vi "Create.vi"(8 "error in (no error)":errorcluster, 9 "offset":i32, 10 "Input":string) -> (0 "error out":errorcluster, 3 "Proto":refnum<class "Proto.lvclass">)   [LabVIEW 2021, in "Proto.lvclass"]
uses:
  Proto.lvclass
  Proto.lvclass/Proto.ctl
  Helpers/Helpers.lvlib
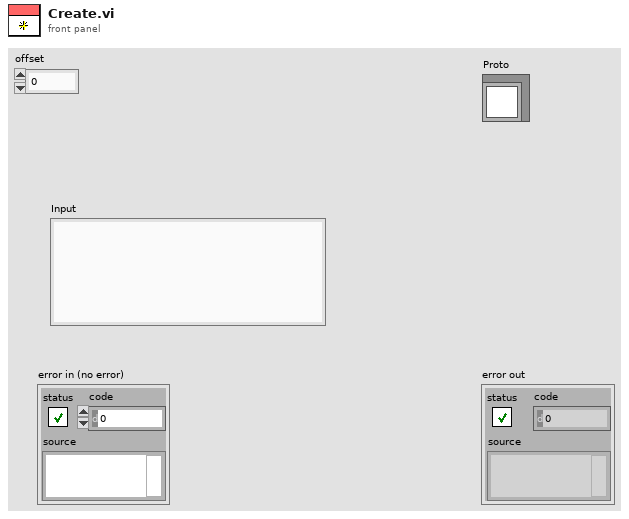
[diagram p1: front panel]
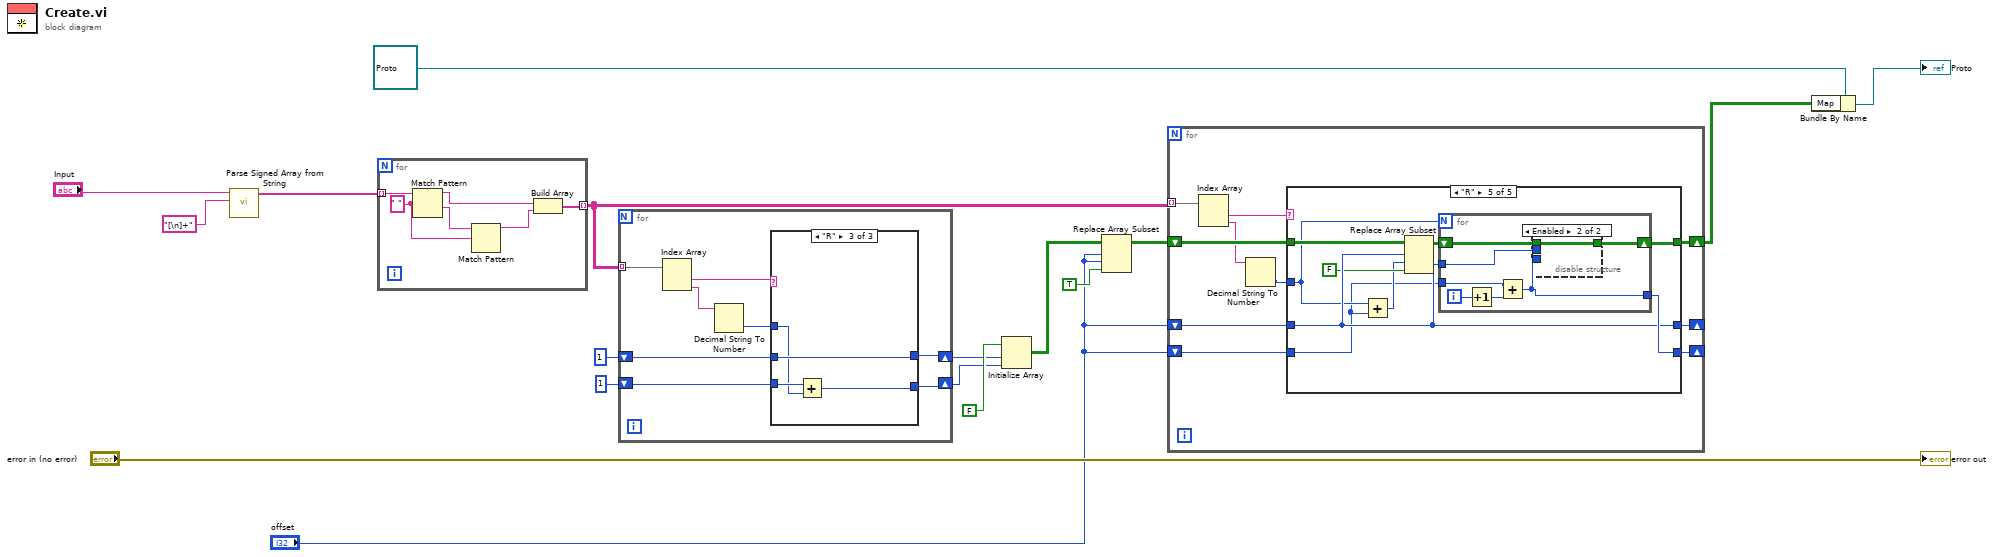
[diagram p0: block diagram]
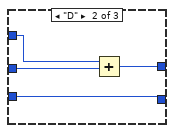
[diagram p3: hidden frame]
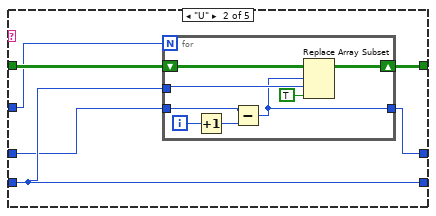
[diagram p5: hidden frame]
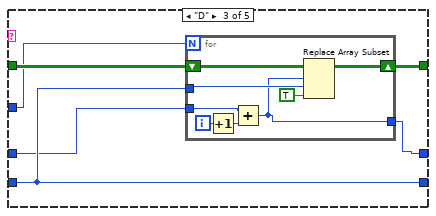
[diagram p6: hidden frame]
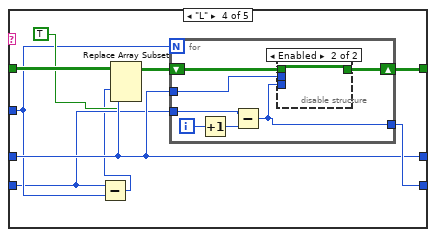
[diagram p7: hidden frame]
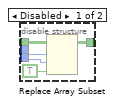
[diagram p8: hidden frame]
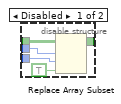
[diagram p9: hidden frame]
diagram:
  n1 = call "Parse Signed Array from String.vi"("Delimiter regex"="[\n]+", "Input"="Input") -> ("Parsed Array"=w13:string[])  [unwired: 8 in, 1 out]
  n2 = for {
    tunnel: w13 -> [w23] mode=indexing
    tunnel: [w18] -> w3 mode=indexing
    w22 = " " ("regular expression")
    n3 = Match Pattern(string=w23, regular expression=w22) -> (before substring=w19:string, after substring=w21:string)  [unwired: 1 in, 2 out]
    n4 = Match Pattern(string=w21, regular expression=w22) -> (before substring=w20:string)  [unwired: 1 in, 3 out]
    n5 = Build Array(w19, w20) -> (w18:string[])
  }
  n6 = for {
    tunnel: w3 -> [w31] mode=indexing
    shift-right: [w24] -> w8
    shift-left: 1 -> [w25]
    shift-right: [w26] -> w9
    shift-left: 1 -> [w27]
    n7 = Index Array(array=w31) -> (element #1=w30:string, element #2=w29:string)  [unwired: 2 in]
    n8 = Decimal String To Number(string=w29) -> (number=w28:i32)  [unwired: 2 in, 1 out]
    n9 = case shown="\"R\"" w30 {
      tunnel: w28 -> [_ w37 w38]
      tunnel: w27 -> [w33 w36 w41]
      tunnel: [w33 w35 w41] -> w26
      tunnel: w25 -> [w32 w34 w40]
      tunnel: [w32 w34 w39] -> w24
      frame Default {
      }
      frame "D" {
        n10 = Add(x=w37, y=w36) -> (x+y=w35:i32)
      }
      frame "R" {
        n11 = Add(x=w40, y=w38) -> (x+y=w39:i32)
      }
    }
  }
  n12 = Initialize Array(FALSE, w9, w8) -> (w6:bool[][])
  n13 = Replace Array Subset(array=w6, new element=TRUE ("new element/subarray"), index (row)="offset", index (col)="offset") -> (w5:bool[][])
  n14 = for {
    tunnel: w3 -> [w51] mode=indexing
    shift-right: [w49] -> w2
    shift-left: w5 -> [w48]
    shift-right: [w45] -> _
    shift-left: "offset" -> [w46]
    shift-right: [w43] -> _
    shift-left: "offset" -> [w44]
    n15 = Index Array(array=w51) -> (element #1=w50:string, element #2=w47:string)  [unwired: 2 in]
    n16 = Decimal String To Number(string=w47) -> (number=w42:i32)  [unwired: 2 in, 1 out]
    n17 = case shown="\"R\"" w50 {
      tunnel: [w54 w58 w72 w90 w112] -> w49
      tunnel: w48 -> [w54 w60 w74 w91 w113]
      tunnel: w46 -> [w53 w56 w70 w87 w109]
      tunnel: [w53 w57 w71 w87 w109] -> w45
      tunnel: w44 -> [w52 w59 w73 w84 w105]
      tunnel: [w52 w59 w73 w89 w111] -> w43
      tunnel: w42 -> [_ w55 w69 w85 w108]
      frame Default {
      }
      frame "U" {
        n18 = for {
          N: w55 -> [_]
          tunnel: w59 -> [w66]
          shift-right: [w67] -> w58
          shift-left: w60 -> [w68]
          tunnel: w56 -> [w64]
          tunnel: [w62] -> w57
          i -> [w65]
          n19 = Increment(x=w65) -> (x+1=w61:i32)
          n20 = Subtract(x=w64, y=w61) -> (x-y=w62:i32)
          n21 = Replace Array Subset(array=w68, new element=TRUE ("new element/subarray"), index (row)=w62, index (col)=w66) -> (w67:bool[][])
        }
      }
      frame "D" {
        n22 = for {
          N: w69 -> [_]
          tunnel: w73 -> [w80]
          shift-right: [w81] -> w72
          shift-left: w74 -> [w82]
          tunnel: w70 -> [w78]
          tunnel: [w76] -> w71
          i -> [w79]
          n23 = Increment(x=w79) -> (x+1=w75:i32)
          n24 = Add(x=w78, y=w75) -> (x+y=w76:i32)
          n25 = Replace Array Subset(array=w82, new element=TRUE ("new element/subarray"), index (row)=w76, index (col)=w80) -> (w81:bool[][])
        }
      }
      frame "L" {
        n26 = Subtract(x=w84, y=w85) -> (x-y=w83:i32)
        n27 = Replace Array Subset(array=w91, new element=TRUE, index (row)=w87, index (col)=w83) -> (w88:bool[][])
        n28 = for {
          N: w85 -> [_]
          tunnel: w87 -> [w93]
          shift-right: [w97] -> w90
          shift-left: w88 -> [w98]
          tunnel: w84 -> [w95]
          tunnel: [w92] -> w89
          i -> [w96]
          n29 = Increment(x=w96) -> (x+1=w94:i32)
          n30 = Subtract(x=w95, y=w94) -> (x-y=w92:i32)
          n31 = disable-structure shown="Enabled" {
            disable-tunnel: w98 -> [w103 w104]
            disable-tunnel: [w102 w104] -> w97
            disable-tunnel: w93 -> [w100 _]
            disable-tunnel: w92 -> [w99 _]
            frame Disabled {
              n32 = Replace Array Subset(array=w103, new element=TRUE ("new element/subarray"), index (row)=w100, index (col)=w99) -> (w102:bool[][])
            }
            frame Enabled {
            }
          }
        }
      }
      frame "R" {
        n33 = Add(x=w108, y=w105) -> (x+y=w106:i32)
        n34 = Replace Array Subset(array=w113, new element=FALSE ("new element/subarray"), index (row)=w109, index (col)=w106) -> (w110:bool[][])
        n35 = for {
          N: w108 -> [_]
          tunnel: w109 -> [w115]
          shift-right: [w119] -> w112
          shift-left: w110 -> [w120]
          tunnel: w105 -> [w117]
          tunnel: [w114] -> w111
          i -> [w118]
          n36 = Increment(x=w118) -> (x+1=w116:i32)
          n37 = Add(x=w117, y=w116) -> (x+y=w114:i32)
          n38 = disable-structure shown="Enabled" {
            disable-tunnel: w120 -> [w125 w126]
            disable-tunnel: [w124 w126] -> w119
            disable-tunnel: w115 -> [w122 _]
            disable-tunnel: w114 -> [w121 _]
            frame Disabled {
              n39 = Replace Array Subset(array=w125, new element=TRUE ("new element/subarray"), index (row)=w122, index (col)=w121) -> (w124:bool[][])
            }
            frame Enabled {
            }
          }
        }
      }
    }
  }
  n40 = Bundle By Name(cluster=refnum<class "Proto.lvclass"> refnum ("Proto"), "Map"=w2) -> (→"Proto":refnum<class "Proto.lvclass">)
  "error out" <- "error in (no error)"
